vi "Write LaserPower Task Name.vi"(8 "error in (no error)":errorcluster, 10 "LaserPower Task Name":refnum<k21>, 11 "AODAcq in":refnum<class "AODAcq.lvclass">) -> (0 "error out":errorcluster, 3 "AODAcq out":refnum<class "AODAcq.lvclass">)   [LabVIEW 2014, in "AODAcq.lvclass"]
uses:
  AODAcq.lvclass
  AODAcq.lvclass/AODAcq.ctl
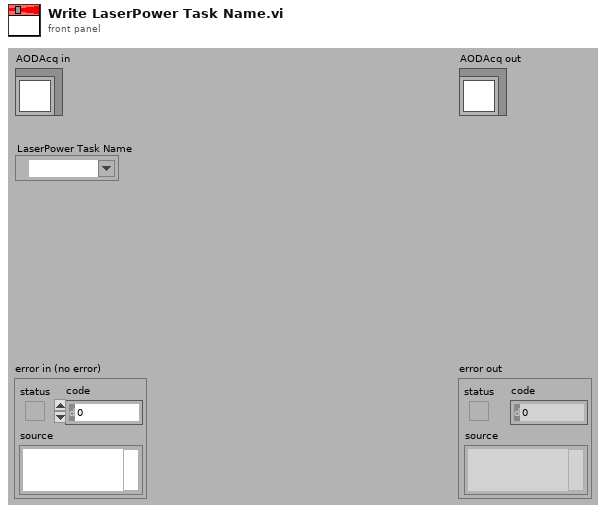
[diagram p1: front panel]
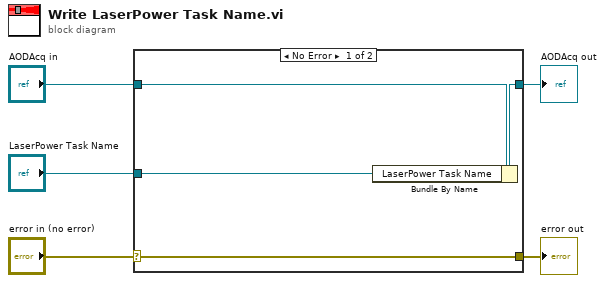
[diagram p0: block diagram]
diagram:
  n1 = case shown="No Error" "error in (no error)" {
    selector: "error in (no error)" -> [w9 w10]
    tunnel: [w9 w10] -> w4
    tunnel: [w7 w11] -> w2
    tunnel: "AODAcq in" -> [w8 w11]
    tunnel: "LaserPower Task Name" -> [w6 _]
    frame No Error {
      n2 = Bundle By Name(cluster=w8, "LaserPower Task Name"=w6) -> (w7:refnum<class "AODAcq.lvclass">)
    }
    frame Error {
    }
  }
  "error out" <- w4
  "AODAcq out" <- w2
